vi "TestArena.vi"() -> ()   [LabVIEW 2013]
uses:
  <vilib>/addons/control/pid/pid.llb/PID Output Rate Limiter (DBL).vi
  <vilib>/addons/control/pid/NI_PID_pid.lvlib
panel:
  out "Elapsed Time (s)":dbl
  in  "Frequency Step Command (Hz)":dbl
  out "Rate Limited Output (Hz)":dbl format="%.2f"
  in  "output rate limit (Hz/s)":dbl=1.0 format="%.2f"
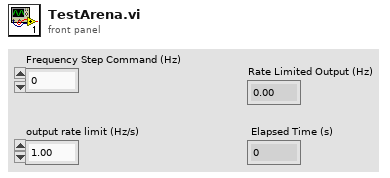
[diagram p1: front panel]
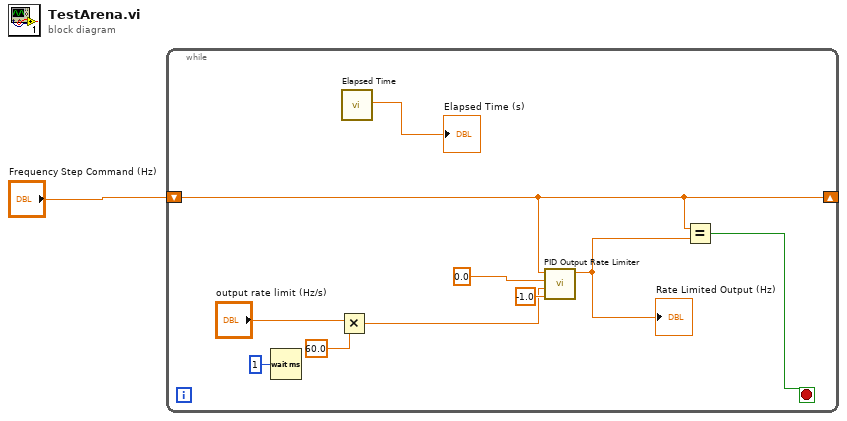
[diagram p0: block diagram]
diagram:
  n1 = while {
    shift-right: [w4] -> _
    shift-left: "Frequency Step Command (Hz)" -> [w4]
    stop <- w3 stop-if-true
    n2 = Wait (ms)(milliseconds to wait=u32 1) -> ()  [unwired: 1 out]
    n3 = Multiply(x="output rate limit (Hz/s)", y=60.0) -> (x*y=w6:dbl)
    n4 = call "Elapsed Time"() -> ("Elapsed Time (s)"=→"Elapsed Time (s)":dbl)  [unwired: 12 in, 7 out]
    n5 = call-poly <vilib>:"PID Output Rate Limiter.vi"("dt (s)"=-1.0, "output rate (EGU/min)"=w6, "initial output"=0.0, "input (controller output)"=w4) -> ("output"=w5:dbl)  [unwired: 4 in, 1 out]
    "Rate Limited Output (Hz)" <- w5
    n6 = Equal?(x=w4, y=w5) -> (x = y?=w3:bool)
  }
